vi "Fix Custom Device Order.vi"(8 "error in":errorcluster, 11 "Device Item Ref in":T1 format="%.0x") -> (0 "error out":errorcluster, 3 "Device Item Ref out":T1 format="%.0x")   [LabVIEW 2017, in "Routing and Faulting System Explorer.lvlib"]
uses:
  Routing and Faulting System Explorer.lvlib
  <vilib>/NI Veristand/Custom Device API/Custom Device Item Ref.ctl
  <vilib>/NI VeriStand/Custom Device API/Custom Device API.lvlib
  Shared/Routing and Faulting Hardware API/Routing and Faulting Hardware API.lvlib
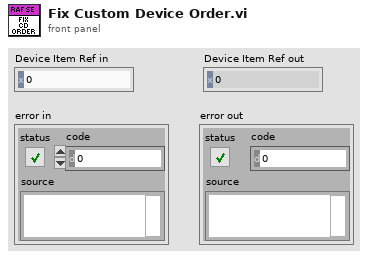
[diagram p1: front panel]
types:
  T1 = typedef "Custom Device API.lvlib/Custom Device Item Ref.ctl" = u64
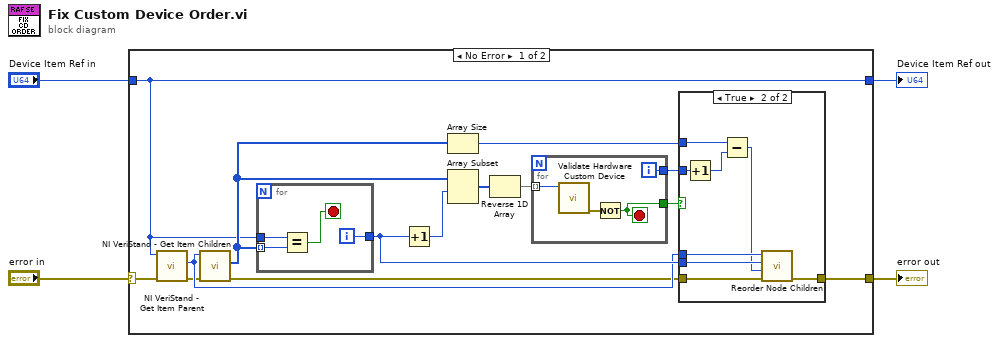
[diagram p0: block diagram]
diagram:
  n1 = case shown="No Error" "error in" {
    selector: "error in" -> [w7 w37]
    tunnel: [w15 w37] -> w4
    tunnel: "Device Item Ref in" -> [w5 w36]
    tunnel: [w5 w36] -> w1
    frame No Error {
      n2 = call <vilib>:"NI VeriStand - Get Item Parent.vi"("error in (no error)"=w7, "Item Ref in"=w5) -> ("error out"=w6:errorcluster, "Parent Ref"=w16:T1)  [unwired: 6 in, 2 out]
      n3 = call <vilib>:"NI VeriStand - Get Item Children.vi"("error in (no error)"=w6, "Item Ref in"=w16) -> ("error out"=w14:errorcluster, "Child Refs"=w18:T1[])  [unwired: 6 in, 2 out]
      n4 = for {
        tunnel: w5 -> [w35]
        tunnel: w18 -> [w34] mode=indexing
        tunnel: [w32] -> w17
        i -> [w32]
        stop <- w33 stop-if-true
        n5 = Equal?(x=w35, y=w34) -> (x = y?=w33:bool)
      }
      n6 = Increment(x=w17) -> (x+1=w9:i32)
      n7 = Array Size(array=w18) -> (size(s)=w11:i32)
      n8 = Array Subset(array=w18, index=w9) -> (w8:T1[])  [unwired: 1 in]
      n9 = Reverse 1D Array(array=w8) -> (reversed array=w10:T1[])
      n10 = for {
        tunnel: w10 -> [w31] mode=indexing
        tunnel: [w29] -> w13
        tunnel: [w28] -> w12
        i -> [w28]
        stop <- w29 stop-if-true
        n11 = call "Validate Hardware Custom Device.vi"("Hardware Ref in"=w31) -> ("error out"=w30:errorcluster)  [unwired: 9 in, 1 out]
        n12 = Not(x=w30) -> (.not. x?=w29:bool)
      }
      n13 = case shown="True" w13 {
        tunnel: w11 -> [_ w27]
        tunnel: w12 -> [_ w26]
        tunnel: w14 -> [w19 w24]
        tunnel: [w19 w23] -> w15
        tunnel: w16 -> [_ w22]
        tunnel: w17 -> [_ w21]
        frame False {
        }
        frame True {
          n14 = Increment(x=w26) -> (x+1=w25:i32)
          n15 = Subtract(x=w27, y=w25) -> (x-y=w20:i32)
          n16 = call "Reorder Node Children.vi"("error in"=w24, "new index"=w20, "current index"=w21, "parent section in"=w22) -> ("error out"=w23:errorcluster)  [unwired: 7 in]
        }
      }
    }
    frame Error {
    }
  }
  "error out" <- w4
  "Device Item Ref out" <- w1
